vi "outline buttons.vi"(9 "control-level":string, 11 "Material-Scheme in":refnum<class "Material-Scheme.lvclass">) -> (1 "font color":u32(colorbox), 2 "colors array":cluster{"bg":u32, "fg":u32}[](array[cluster]))   [LabVIEW 2021, in "TSC Material Theme.lvlib" / "Material-Scheme.lvclass"]
doc: "application of the OUTLINE buttons coloring rules\n\n-->this VI is <i>public</i> because it is used in the Button Editor UI\n\nhttps://m3.material.io/components/buttons/specs#6757c97e-0ae6-4802-a2d5-9e3b134a7231\n\n<b>Code Developed By:</b>\nTechnology Service Corporation\nwww.tsc.com/atcs\n\nDeveloper:\nDaniel Coons"
uses:
  Material-Scheme.lvclass
  <vilib>/Utility/colorconv.llb/Color to RGB.vi
  <vilib>/Utility/colorconv.llb/RGB to Color.vi
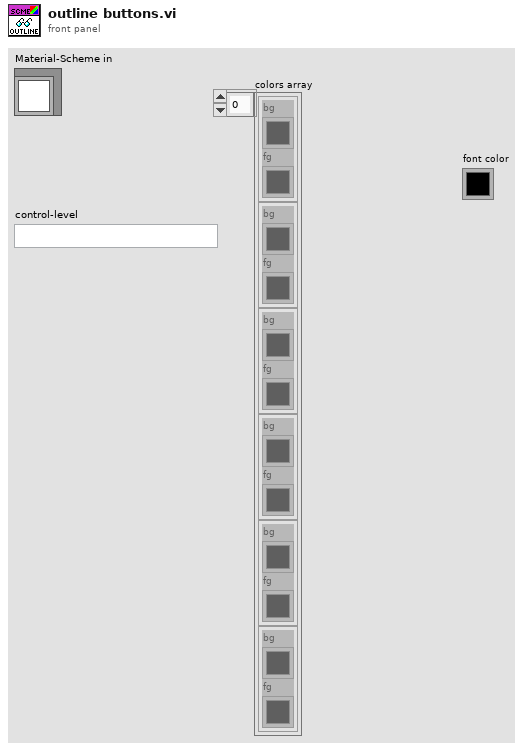
[diagram p1: front panel]
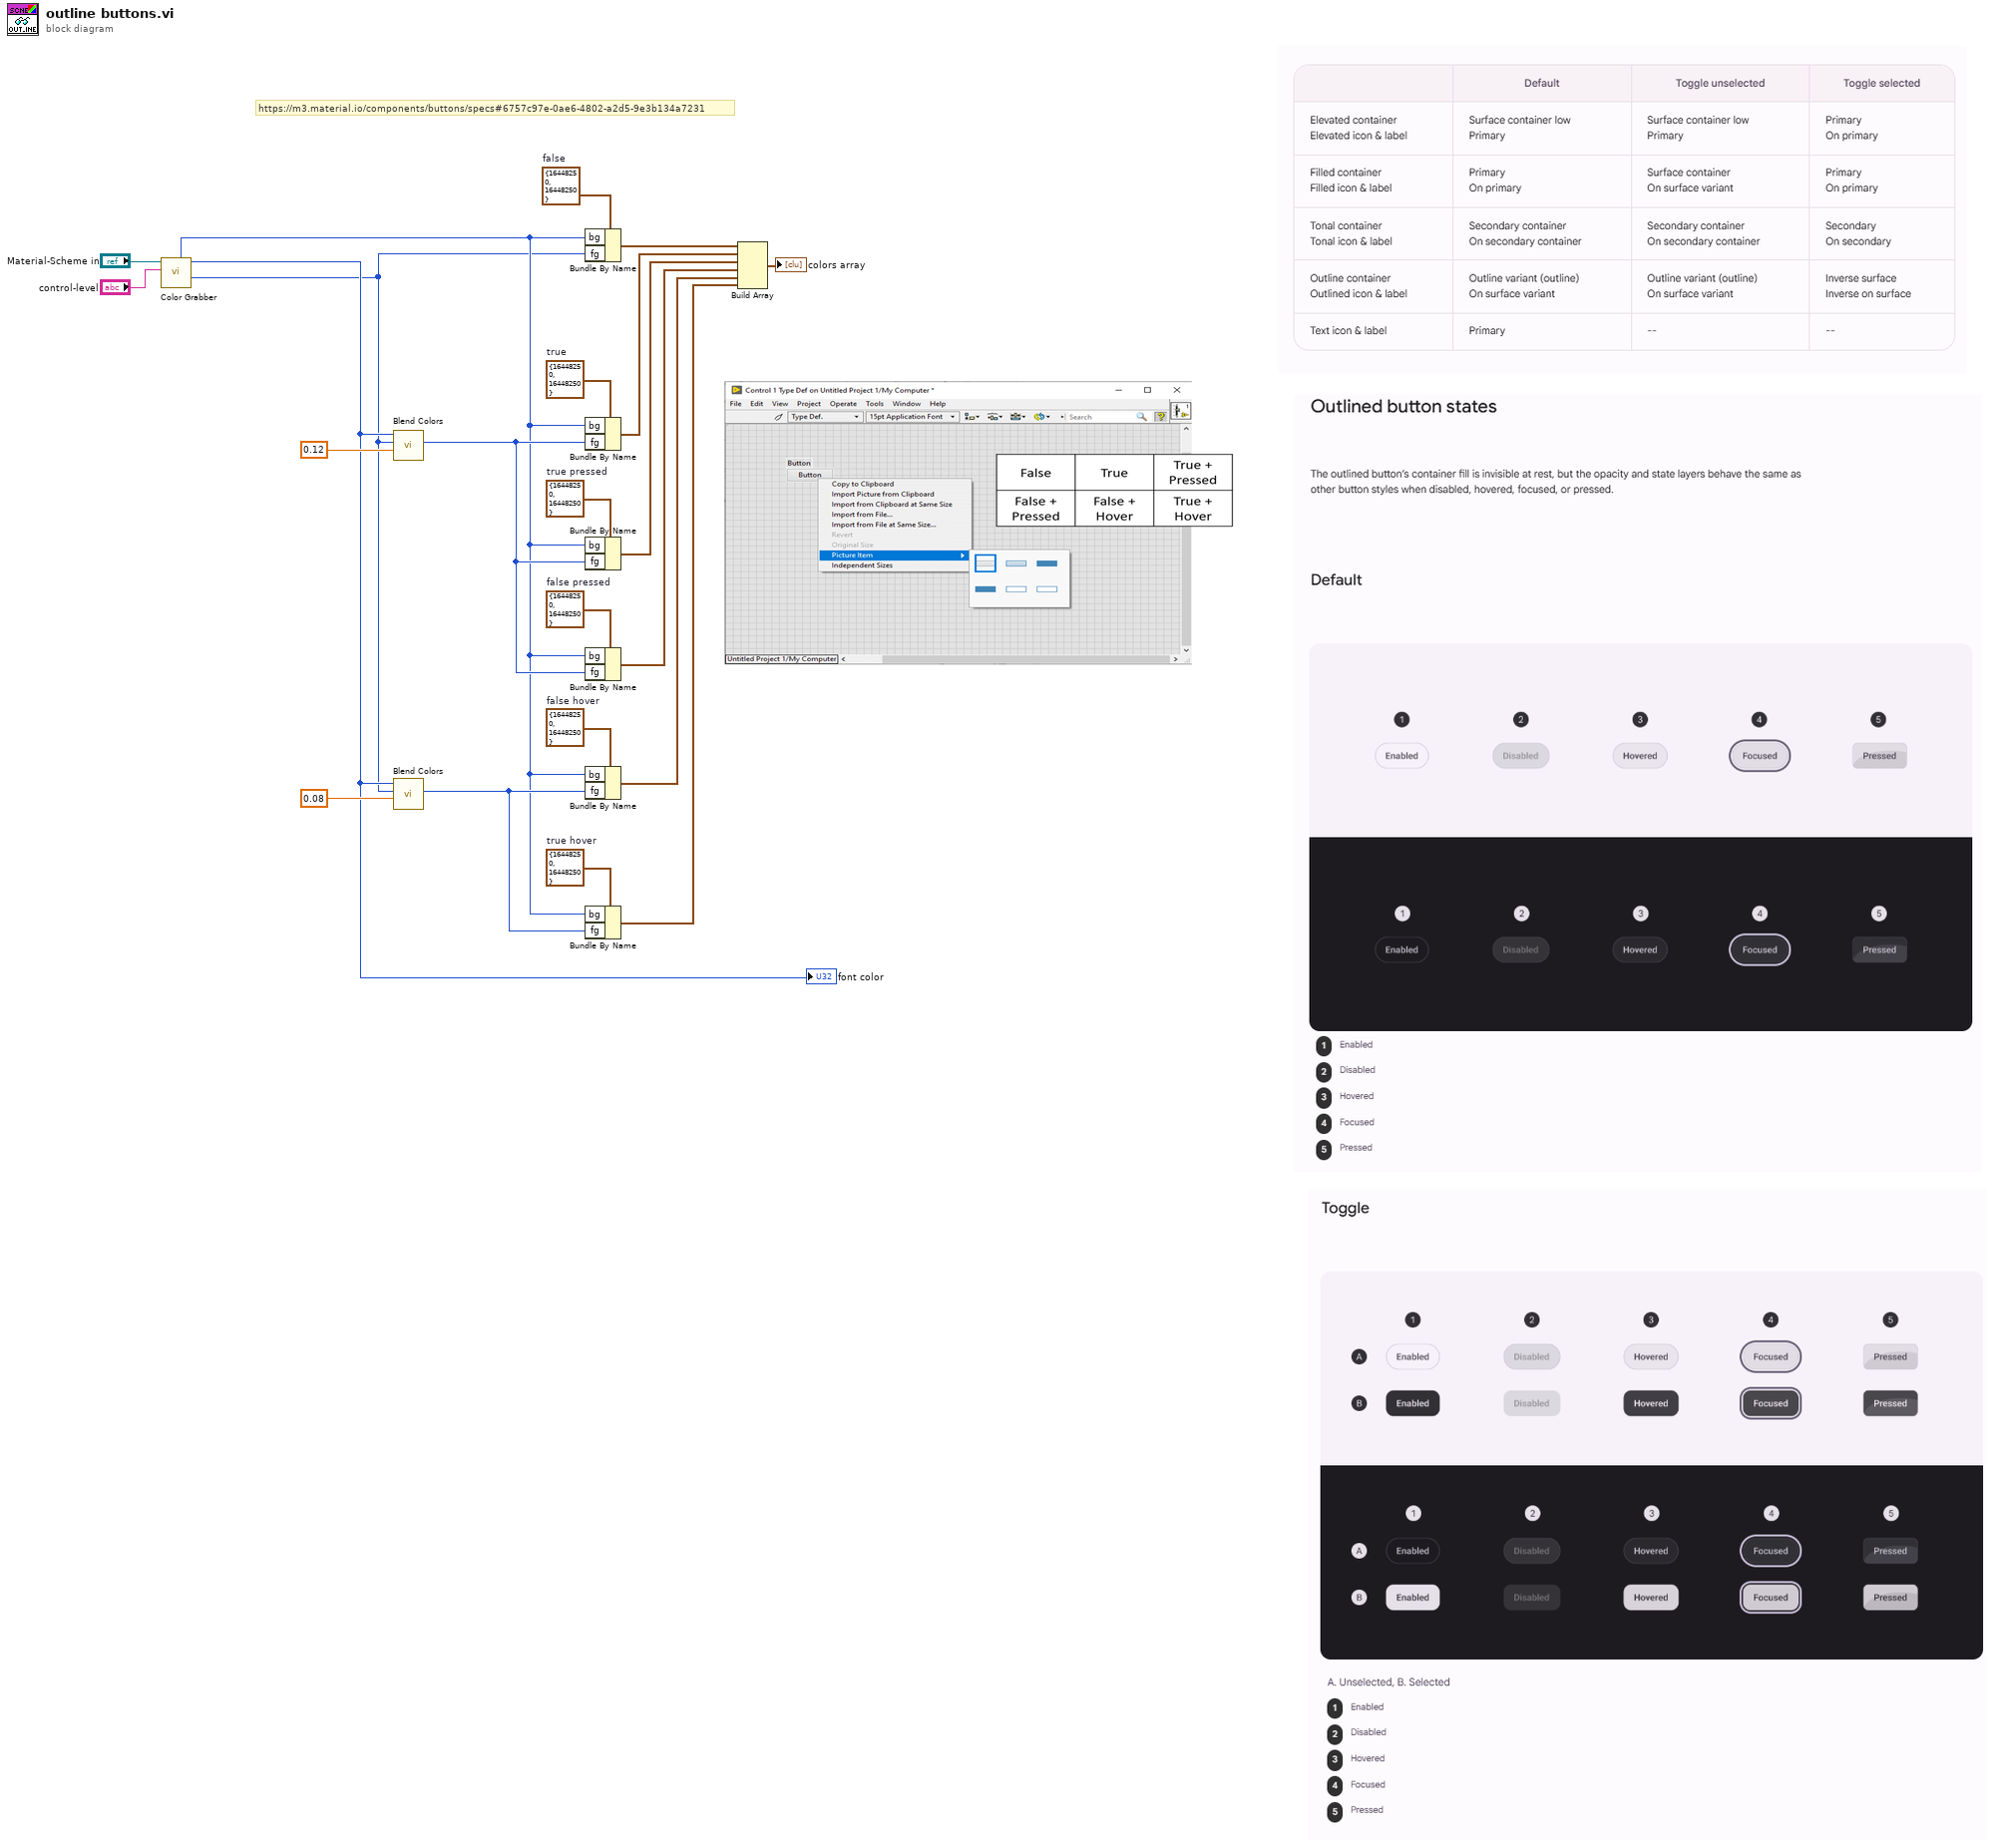
[diagram p0: block diagram]
diagram:
  w17 = cluster{"bg":u32, "fg":u32} {"bg"=16448250, "fg"=16448250}  # true hover
  w18 = cluster{"bg":u32, "fg":u32} {"bg"=16448250, "fg"=16448250}  # false hover
  w19 = cluster{"bg":u32, "fg":u32} {"bg"=16448250, "fg"=16448250}  # false pressed
  w20 = cluster{"bg":u32, "fg":u32} {"bg"=16448250, "fg"=16448250}  # true pressed
  w21 = cluster{"bg":u32, "fg":u32} {"bg"=16448250, "fg"=16448250}  # true
  w22 = cluster{"bg":u32, "fg":u32} {"bg"=16448250, "fg"=16448250}  # false
  # "https://m3.material.io/components/buttons/specs#6757c97e-0ae6-4802-a2d5-9e3b134a7231"
  n1 = call "Color Grabber.vi"("control-level"="control-level", "Material-Scheme in"="Material-Scheme in") -> ("surface"=w1:u32, "color"=w2:u32, "outline"=w3:u32)  [unwired: 3 in, 4 out]
  "font color" <- w2
  n2 = call "Blend Colors.vi"("blend ratio"=0.12, "onColor"=w1, "Color"=w2) -> ("Modified Color"=w4:u32)  [unwired: 8 in]
  n3 = call "Blend Colors.vi"("blend ratio"=0.08, "onColor"=w1, "Color"=w2) -> ("Modified Color"=w7:u32)  [unwired: 8 in]
  n4 = Bundle By Name(cluster=w22, "bg"=w3, "fg"=w1) -> (w16:cluster{"bg":u32, "fg":u32})
  n5 = Bundle By Name(cluster=w21, "bg"=w3, "fg"=w4) -> (w15:cluster{"bg":u32, "fg":u32})
  n6 = Bundle By Name(cluster=w20, "bg"=w3, "fg"=w4) -> (w14:cluster{"bg":u32, "fg":u32})
  n7 = Bundle By Name(cluster=w19, "bg"=w3, "fg"=w4) -> (w13:cluster{"bg":u32, "fg":u32})
  n8 = Bundle By Name(cluster=w18, "bg"=w3, "fg"=w7) -> (w12:cluster{"bg":u32, "fg":u32})
  n9 = Bundle By Name(cluster=w17, "bg"=w3, "fg"=w7) -> (w11:cluster{"bg":u32, "fg":u32})
  n10 = Build Array(w16, w15, w14, w13, w12, w11) -> (→"colors array":cluster{"bg":u32, "fg":u32}[])
